vi "Select Worksheet by Index.vi"(2 "error in (no error)":errorcluster, 3 "Worksheet Index":i32, 4 "Report Ref In":T1) -> (0 "error out":errorcluster, 1 "Report Ref Out":T1)   [LabVIEW 2013, in "XCel Report Engine.lvlib"]
doc: "Selects a worksheet by its zero-based index and makes it the active worksheet for subsequent report operations.\n\nIndex 0 selects the first worksheet in workbook order.\n\nAn error is returned if the index is negative or outside the available worksheet range."
uses:
  XCel Report Engine.lvlib
  C:/Users/m.santucci/Documents/ChatGPT/LV_REPORT_ENGINE/LV/DotNet/XCelReportEngine.dll
  LV/DotNet/XCelReportEngine.dll
  Controls/Report Ref.ctl
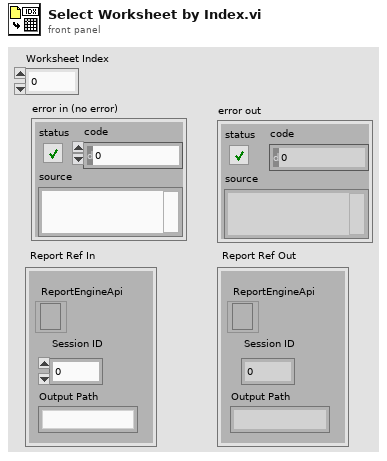
[diagram p1: front panel]
types:
  T1 = typedef "XCel Report Engine.lvlib/Report Ref.ctl" = cluster{"Session ID":i32, "Output Path":string, "ReportEngineApi":refnum<k24>}
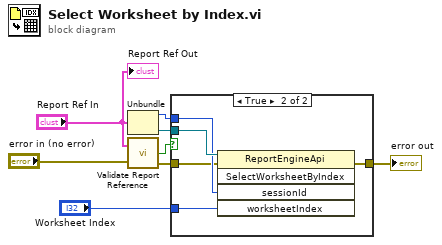
[diagram p0: block diagram]
diagram:
  n1 = Unbundle("Report Ref In") -> ("Session ID"=w7:i32, "ReportEngineApi"=w8:refnum<k24>)  [unwired: 1 out]
  n2 = call "Validate Report Reference.vi"("Report Ref In"="Report Ref In", "error in (no error)"="error in (no error)") -> ("Valid"=w1:bool, "error out"=w2:errorcluster)  [unwired: 1 out]
  n3 = case shown="True" w1 {
    tunnel: w8 -> [_ w14]
    tunnel: w7 -> [_ w13]
    tunnel: "Worksheet Index" -> [_ w12]
    tunnel: [w9 w11] -> w5
    tunnel: w2 -> [w9 w10]
    frame False {
    }
    frame True {
      n4 = invoke class="ReportEngineApi" method="SelectWorksheetByIndex"(reference=w14, error in=w10, "sessionId"=w13, "worksheetIndex"=w12) -> (error out=w11:errorcluster)  [unwired: 1 in, 4 out]
    }
  }
  "error out" <- w5
  "Report Ref Out" <- "Report Ref In"
